vi "CoilConfig.vi"(0 "Card Info":cluster{"Card Handle":u32, "Error Code":u32}, 1 "AO Channels":i32, 2 "Stop angle [deg]":dbl=8.0 min=0.75 max=16.7 step=0.01 format="%.2g", 5 "Frequency (Hz)":dbl, 7 "Field [mT]":dbl=8.0 min=0.75 max=16.7 step=0.01 format="%.2g", 9 "Bit Resolution":i32, 11 "Clamp field [%]":sgl, 12 "Number of Turns":dbl) -> ()   [LabVIEW 2011]
uses:
  spcm_library/spcm_card.llb/setup DO/AO trigger.vi
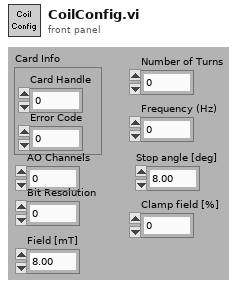
[diagram p1: front panel]
types:
  T1 = cluster{"Enable":bool, "Offs":i32, "Gain":i32, "Filter":i32, "Output Mode":u16}
  T2 = cluster{"Trig Termination":bool, "Trigger Source":u16, "External Trigger":u16, "Ext Pw":u32, "Trigger Delay (Samples)":u32, "Trig Output":bool}
  T3 = cluster{"Mode":u16, "Mem":u32, "Seg":u32, "Loop":u32}
  T4 = cluster{"Clock Mode":u16, "Sampling Rate (kHz)":i32, "Reference Clock (kHz)":i32, "Clock Output":bool, "Clock Termination":bool, "External Divider":i32}
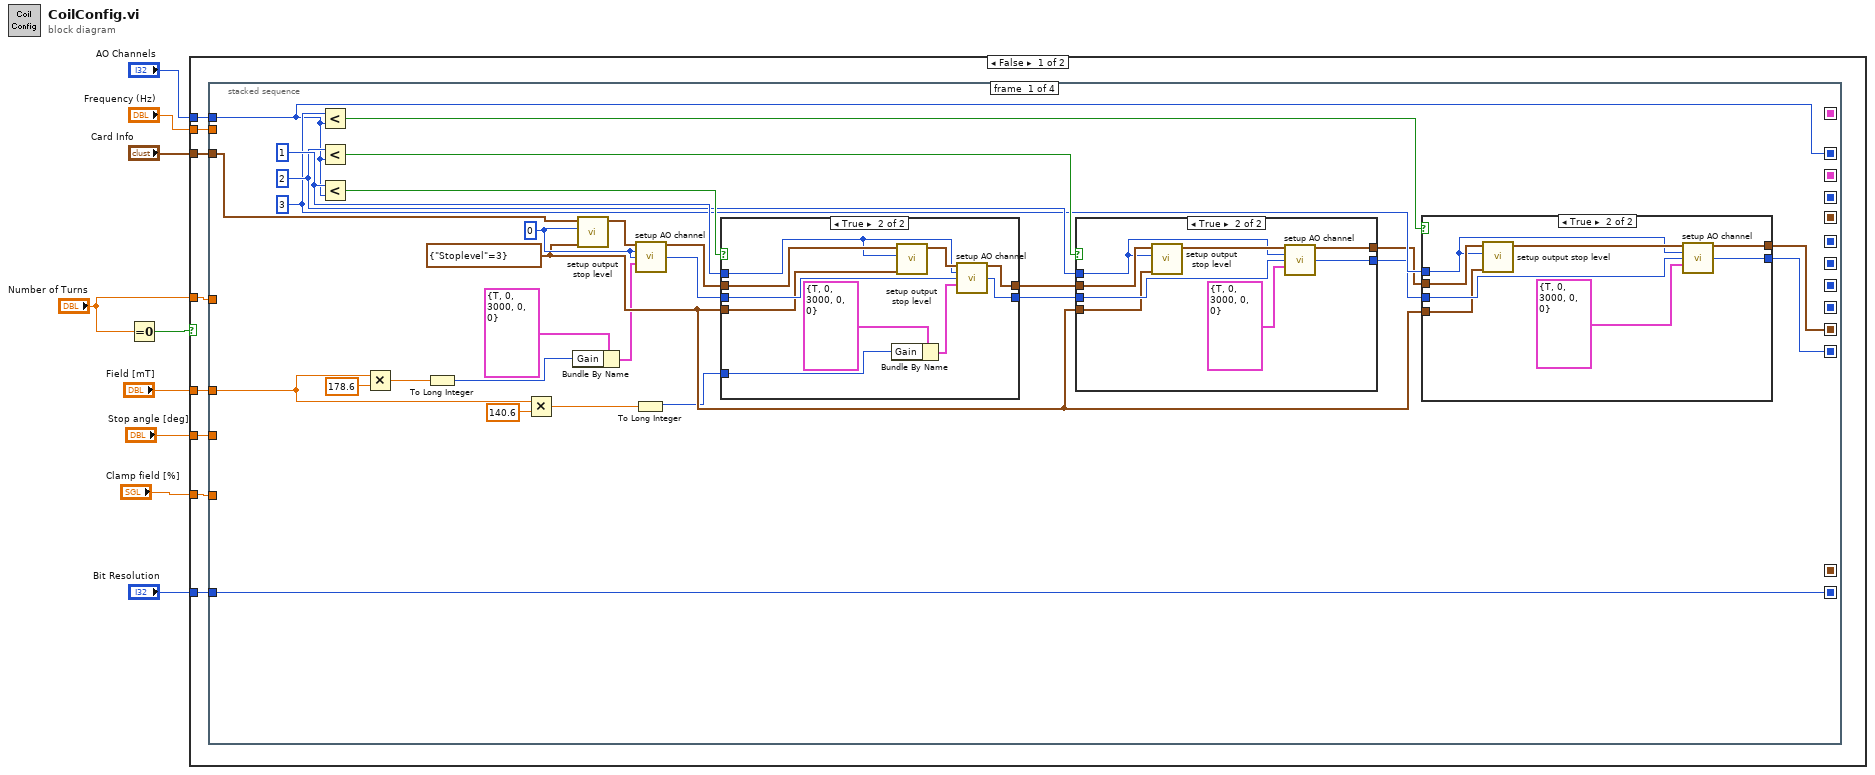
[diagram p0: block diagram]
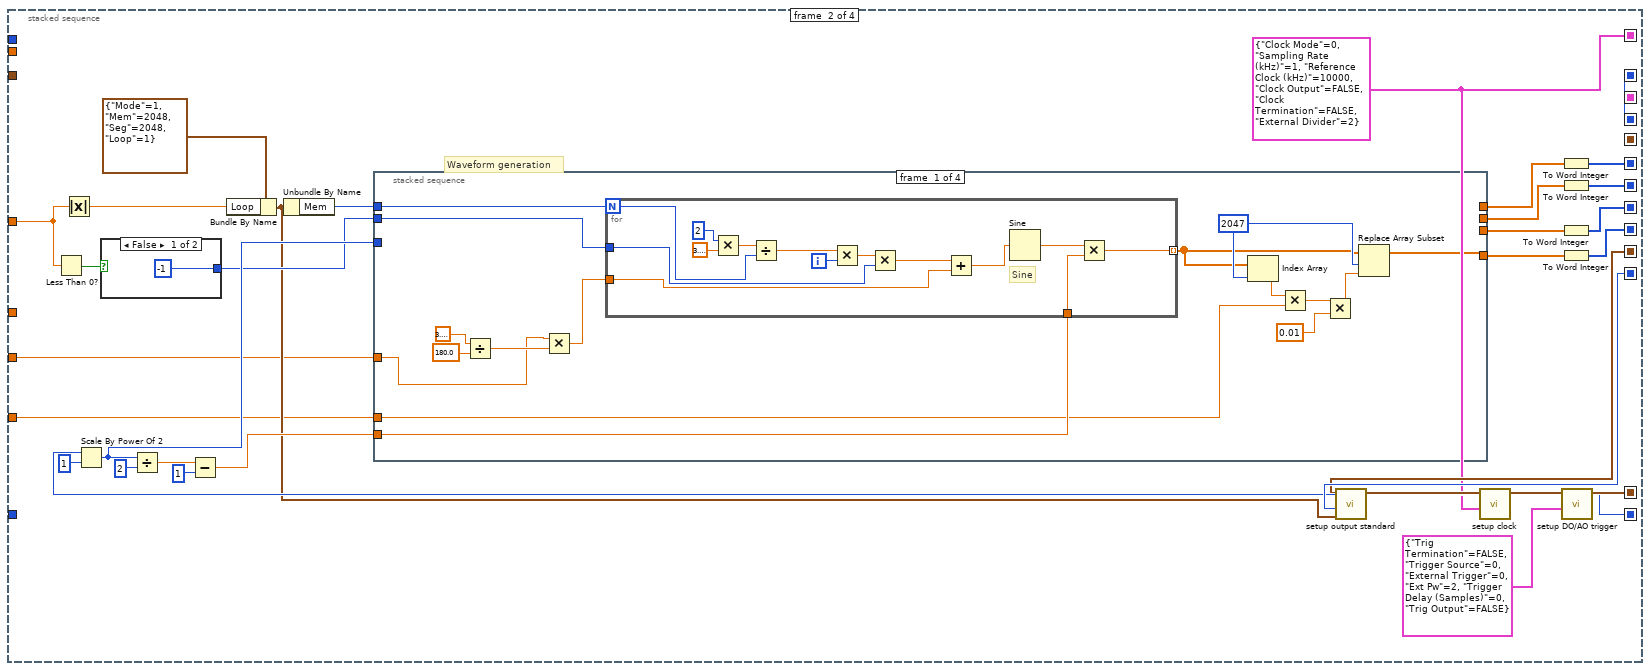
[diagram p5: hidden frame]
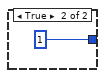
[diagram p6: hidden frame]
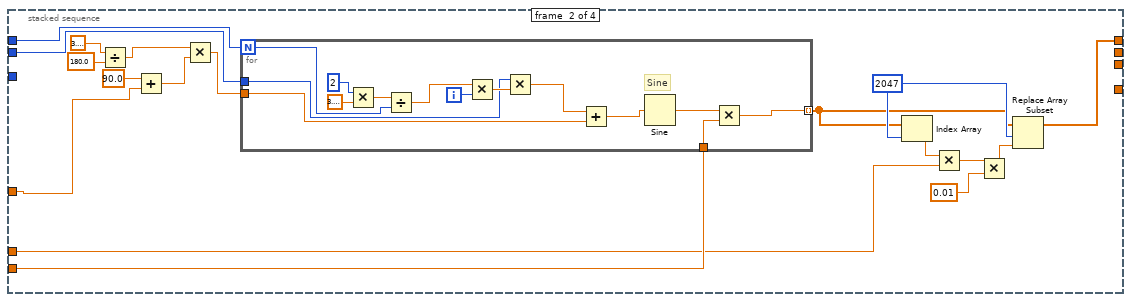
[diagram p7: hidden frame]
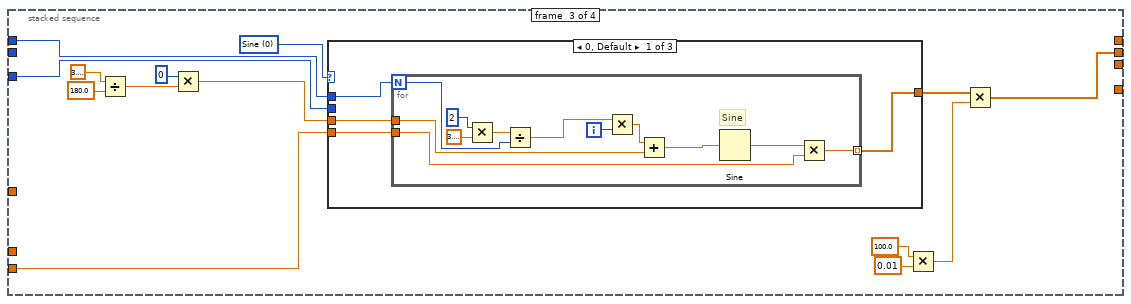
[diagram p8: hidden frame]
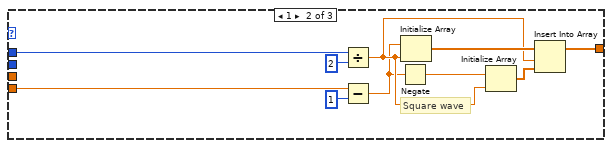
[diagram p9: hidden frame]
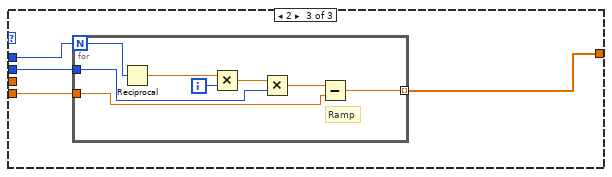
[diagram p10: hidden frame]
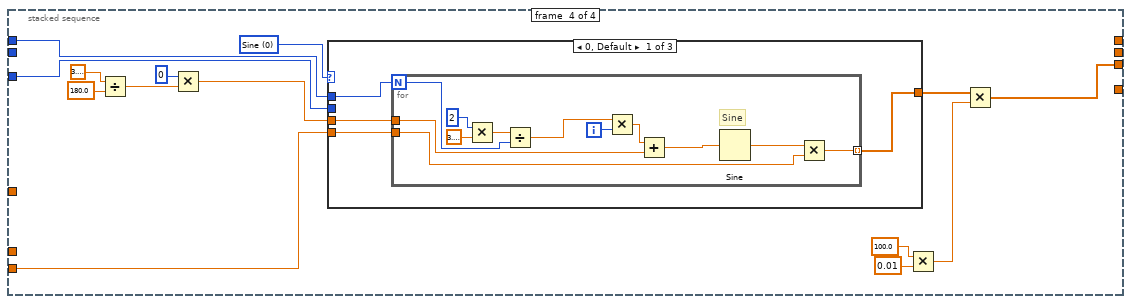
[diagram p11: hidden frame]
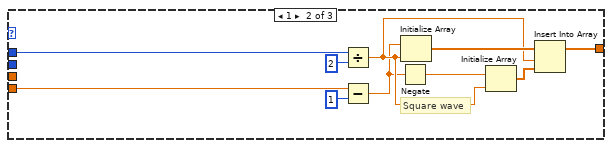
[diagram p12: hidden frame]
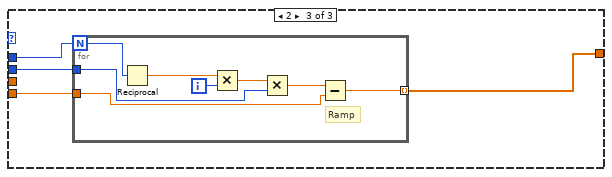
[diagram p13: hidden frame]
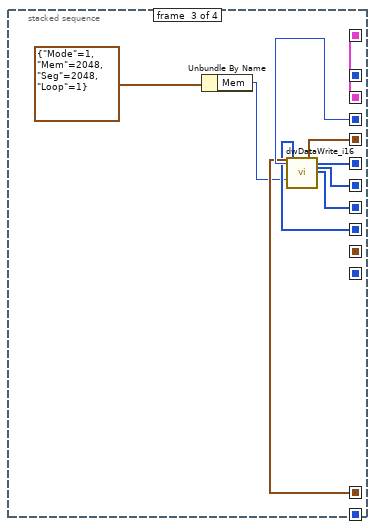
[diagram p14: hidden frame]
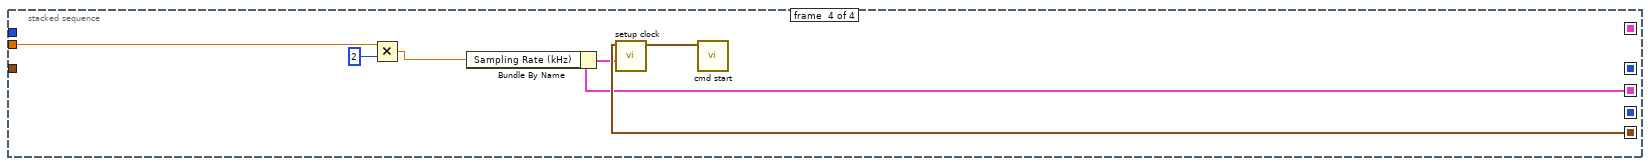
[diagram p15: hidden frame]
diagram:
  n1 = Equal To 0?(x="Number of Turns") -> (x = 0?=w3:bool)
  n2 = case shown="False" w3 {
    tunnel: "Frequency (Hz)" -> [w17 _]
    tunnel: "Clamp field [%]" -> [w16 _]
    tunnel: "Card Info" -> [w15 _]
    tunnel: "Number of Turns" -> [w14 _]
    tunnel: "Bit Resolution" -> [w13 _]
    tunnel: "AO Channels" -> [w12 _]
    tunnel: "Field [mT]" -> [w11 _]
    tunnel: "Stop angle [deg]" -> [w10 _]
    frame False {
      n3 = stacked-sequence {
        seq-local: [w29 _ _ _] -> [_ w104 _ _]
        seq-local: [w31 _ _ _] -> [_ w84 _ _]
        seq-local: [w44 _ _ _] -> [_ w102 _ _]
        seq-local: [w30 _ _ _] -> [_ w106 _ _]
        seq-local: [_ w88 _ _] -> [_ _ w280 _]
        seq-local: [_ w84 _ _] -> [_ _ w288 _]
        seq-local: [_ w108 _ _] -> [_ _ w287 _]
        seq-local: [_ w100 _ _] -> [_ _ w283 _]
        seq-local: [_ w99 _ _] -> [_ _ w284 _]
        seq-local: [_ w98 _ _] -> [_ _ w285 _]
        seq-local: [_ w97 _ _] -> [_ _ w286 _]
        seq-local: [_ _ w281 _] -> [_ _ _ w294]
        seq-local: [_ _ w280 _] -> [_ _ _ w293]
        tunnel: w13 -> [w29 _ _ _]
        tunnel: w12 -> [w31 _ _ _]
        tunnel: w15 -> [w28 _ _ _]
        tunnel: w16 -> [_ w83 _ _]
        tunnel: w14 -> [_ w81 _ _]
        tunnel: w17 -> [_ _ _ w290]
        tunnel: w11 -> [w18 _ _ _]
        tunnel: w10 -> [_ w79 _ _]
        frame #0 {
          w23 = cluster{"Stoplevel":u16} {"Stoplevel"=3} ("Stop Level")
          w36 = 3
          w38 = 2
          w45 = 1
          w42 = 0
          n4 = Less?(x=w36, y=w31) -> (x < y?=w37:bool)
          n5 = Less?(x=w38, y=w31) -> (x < y?=w39:bool)
          n6 = Less?(x=w45, y=w31) -> (x < y?=w46:bool)
          n7 = Multiply(x=w18, y=178.6) -> (x*y=w26:dbl)
          n8 = To Long Integer(number=w26) -> (32bit integer=w20:i32)
          n9 = Multiply(x=w18, y=140.6) -> (x*y=w25:dbl)
          n10 = Bundle By Name(cluster=T1 {"Enable"=TRUE, "Offs"=0, "Gain"=3000, "Filter"=0, "Output Mode"=0} ("Input Channel Settings"), "Gain"=w20) -> (w21:T1)
          n11 = call "setup output stop level.vi"("Stop Level"=w23, "Index"=w42, "Card Info In"=w28) -> ("Card Info Out"=w43:cluster{"Card Handle":u32, "Error Code":u32})  [unwired: 4 in]
          n12 = To Long Integer(number=w25) -> (32bit integer=w19:i32)
          n13 = call "setup AO channel.vi"("Card Info In"=w43, "Channel Index"=w42, "Channel Mask In"=w42, "Input Channel Settings"=w21) -> ("Card Info Out"=w41:cluster{"Card Handle":u32, "Error Code":u32}, "Channel MaskOut"=w40:i32)  [unwired: 10 in]
          n14 = case shown="True" w46 {
            tunnel: [w68 w76] -> w35
            tunnel: w41 -> [w68 w78]
            tunnel: w45 -> [_ w74]
            tunnel: w40 -> [w67 w75]
            tunnel: w23 -> [_ w73]
            tunnel: [w67 w72] -> w33
            tunnel: w19 -> [_ w69]
            frame False {
            }
            frame True {
              n15 = Bundle By Name(cluster=T1 {"Enable"=TRUE, "Offs"=0, "Gain"=3000, "Filter"=0, "Output Mode"=0} ("Input Channel Settings 2"), "Gain"=w69) -> (w71:T1)
              n16 = call "setup output stop level.vi"("Stop Level"=w73, "Index"=w74, "Card Info In"=w78) -> ("Card Info Out"=w77:cluster{"Card Handle":u32, "Error Code":u32})  [unwired: 4 in]
              n17 = call "setup AO channel.vi"("Card Info In"=w77, "Channel Index"=w74, "Channel Mask In"=w75, "Input Channel Settings"=w71) -> ("Card Info Out"=w76:cluster{"Card Handle":u32, "Error Code":u32}, "Channel MaskOut"=w72:i32)  [unwired: 10 in]
            }
          }
          n18 = case shown="True" w39 {
            tunnel: [w58 w64] -> w34
            tunnel: w35 -> [w58 w66]
            tunnel: w38 -> [_ w62]
            tunnel: w33 -> [w57 w63]
            tunnel: w23 -> [_ w61]
            tunnel: [w57 w60] -> w32
            frame False {
            }
            frame True {
              n19 = call "setup output stop level.vi"("Stop Level"=w61, "Index"=w62, "Card Info In"=w66) -> ("Card Info Out"=w65:cluster{"Card Handle":u32, "Error Code":u32})  [unwired: 4 in]
              n20 = call "setup AO channel.vi"("Card Info In"=w65, "Channel Index"=w62, "Channel Mask In"=w63, "Input Channel Settings"=T1 {"Enable"=TRUE, "Offs"=0, "Gain"=3000, "Filter"=0, "Output Mode"=0} ("Input Channel Settings 3")) -> ("Card Info Out"=w64:cluster{"Card Handle":u32, "Error Code":u32}, "Channel MaskOut"=w60:i32)  [unwired: 10 in]
            }
          }
          n21 = case shown="True" w37 {
            tunnel: [w48 w54] -> w44
            tunnel: w34 -> [w48 w56]
            tunnel: w36 -> [_ w52]
            tunnel: w32 -> [w47 w53]
            tunnel: w23 -> [_ w51]
            tunnel: [w47 w50] -> w30
            frame False {
            }
            frame True {
              n22 = call "setup output stop level.vi"("Stop Level"=w51, "Index"=w52, "Card Info In"=w56) -> ("Card Info Out"=w55:cluster{"Card Handle":u32, "Error Code":u32})  [unwired: 4 in]
              n23 = call "setup AO channel.vi"("Card Info In"=w55, "Channel Index"=w52, "Channel Mask In"=w53, "Input Channel Settings"=T1 {"Enable"=TRUE, "Offs"=0, "Gain"=3000, "Filter"=0, "Output Mode"=0} ("Input Channel Settings 4")) -> ("Card Info Out"=w54:cluster{"Card Handle":u32, "Error Code":u32}, "Channel MaskOut"=w50:i32)  [unwired: 10 in]
            }
          }
        }
        frame #1 {
          w88 = T4 {"Clock Mode"=0, "Sampling Rate (kHz)"=1, "Reference Clock (kHz)"=10000, "Clock Output"=FALSE, "Clock Termination"=FALSE, "External Divider"=2} ("Clock Settings")
          # "Waveform generation"
          n24 = Less Than 0?(x=w81) -> (x < 0?=w82:bool)
          n25 = Absolute Value(x=w81) -> (abs(x)=w80:dbl)
          n26 = Scale By Power Of 2(n=w104, x=1) -> (x*2^n=w89:i32)
          n27 = case shown="False" w82 {
            tunnel: [i16 -1 ("Phase 3") i16 1 ("Phase 3")] -> w87
            frame False {
            }
            frame True {
            }
          }
          n28 = Divide(x=w89, y=2) -> (x/y=w90:dbl)
          n29 = Subtract(x=w90, y=1) -> (x-y=w92:dbl)
          n30 = Bundle By Name(cluster=T3 {"Mode"=1, "Mem"=2048, "Seg"=2048, "Loop"=1} ("Mode Setup"), "Loop"=w80) -> (w85:T3)
          n31 = Unbundle By Name(w85) -> ("Mem"=w103:u32)
          n32 = stacked-sequence {
            tunnel: [w115 _ _ _] -> w101
            tunnel: w103 -> [w128 w160 w182 w234]
            tunnel: [_ w145 _ _] -> w96
            tunnel: [_ _ w185 _] -> w95
            tunnel: [_ _ _ w237] -> w94
            tunnel: w92 -> [w127 w159 w181 w233]
            tunnel: w89 -> [_ _ w180 w232]
            tunnel: w87 -> [w122 w155 _ _]
            tunnel: w83 -> [w113 w143 _ _]
            tunnel: w79 -> [w121 w151 _ _]
            frame #0 {
              w120 = 2047 ("index")
              n33 = Divide(x=3.141592653589793, y=sgl 180.0 ("Numeric")) -> (x/y=w124:dbl)
              n34 = Multiply(x=w121, y=w124) -> (x*y=w123:dbl)
              n35 = for {
                N: w128 -> [w136]
                tunnel: [w132] -> w114 mode=indexing
                tunnel: w127 -> [w141]
                tunnel: w123 -> [w134]
                tunnel: w122 -> [w129]
                i -> [w137]
                # "Sine"
                n36 = Multiply(x=2, y=3.141592653589793) -> (x*y=w135:dbl)
                n37 = Divide(x=w135, y=w136) -> (x/y=w138:dbl)
                n38 = Multiply(x=w138, y=w137) -> (x*y=w131:dbl)
                n39 = Multiply(x=w131, y=w129) -> (x*y=w130:dbl)
                n40 = Add(x=w130, y=w134) -> (x+y=w133:dbl)
                n41 = Sine(x=w133) -> (sin(x)=w142:dbl)
                n42 = Multiply(x=w142, y=w141) -> (x*y=w132:dbl)
              }
              n43 = Index Array(array=w114, index=w120) -> (element=w116:dbl)
              n44 = Multiply(x=w116, y=w113) -> (x*y=w119:dbl)
              n45 = Multiply(x=w119, y=0.01) -> (x*y=w117:dbl)
              n46 = Replace Array Subset(array=w114, new element=w117, index=w120) -> (w115:dbl[])
            }
            frame #1 {
              w150 = 2047 ("index")
              n47 = Divide(x=3.141592653589793, y=sgl 180.0 ("Numeric")) -> (x/y=w154:dbl)
              n48 = Add(x=90.0, y=w151) -> (x+y=w153:dbl)
              n49 = Multiply(x=w154, y=w153) -> (x*y=w156:dbl)
              n50 = for {
                N: w160 -> [w168]
                tunnel: [w166] -> w144 mode=indexing
                tunnel: w159 -> [w173]
                tunnel: w156 -> [w164]
                tunnel: w155 -> [w161]
                i -> [w169]
                # "Sine"
                n51 = Multiply(x=2, y=3.141592653589793) -> (x*y=w167:dbl)
                n52 = Divide(x=w167, y=w168) -> (x/y=w170:dbl)
                n53 = Multiply(x=w170, y=w169) -> (x*y=w162:dbl)
                n54 = Multiply(x=w161, y=w162) -> (x*y=w163:dbl)
                n55 = Add(x=w163, y=w164) -> (x+y=w165:dbl)
                n56 = Sine(x=w165) -> (sin(x)=w174:dbl)
                n57 = Multiply(x=w174, y=w173) -> (x*y=w166:dbl)
              }
              n58 = Index Array(array=w144, index=w150) -> (element=w146:dbl)
              n59 = Multiply(x=w146, y=w143) -> (x*y=w149:dbl)
              n60 = Multiply(x=w149, y=0.01) -> (x*y=w147:dbl)
              n61 = Replace Array Subset(array=w144, new element=w147, index=w150) -> (w145:dbl[])
            }
            frame #2 {
              w183 = u16 0 items=["Sine", "Square", "Ramp"] ("Waveform 3")
              n62 = Divide(x=3.141592653589793, y=sgl 180.0 ("Numeric")) -> (x/y=w177:dbl)
              n63 = Multiply(x=i16 0 ("Phase"), y=w177) -> (x*y=w176:dbl)
              n64 = case shown="0, Default" w183 {
                tunnel: w182 -> [w192 w214 w218]
                tunnel: [w191 w210 w217] -> w184
                tunnel: w181 -> [w190 w205 w216]
                tunnel: w180 -> [_ _ w215]
                tunnel: w176 -> [w189 _ _]
                frame 0, Default {
                  n65 = for {
                    N: w192 -> [w198]
                    tunnel: [w196] -> w191 mode=indexing
                    tunnel: w190 -> [w203]
                    tunnel: w189 -> [w193]
                    i -> [w199]
                    # "Sine"
                    n66 = Multiply(x=2, y=3.141592653589793) -> (x*y=w197:dbl)
                    n67 = Divide(x=w197, y=w198) -> (x/y=w200:dbl)
                    n68 = Multiply(x=w200, y=w199) -> (x*y=w194:dbl)
                    n69 = Add(x=w194, y=w193) -> (x+y=w195:dbl)
                    n70 = Sine(x=w195) -> (sin(x)=w204:dbl)
                    n71 = Multiply(x=w204, y=w203) -> (x*y=w196:dbl)
                  }
                }
                frame 1 {
                  # "Square wave"
                  n72 = Divide(x=w214, y=2) -> (x/y=w209:dbl)
                  n73 = Subtract(x=w205, y=1) -> (x-y=w207:dbl)
                  n74 = Negate(x=w207) -> (-x=w208:dbl)
                  n75 = Initialize Array(w207, w209) -> (w212:dbl[])
                  n76 = Initialize Array(w208, w209) -> (w211:dbl[])
                  n77 = Insert Into Array(array=w212, index=w209, new element=w211) -> (w210:dbl[])
                }
                frame 2 {
                  n78 = for {
                    N: w218 -> [w221]
                    tunnel: [w223] -> w217 mode=indexing
                    tunnel: w216 -> [w220]
                    tunnel: w215 -> [w219]
                    i -> [w225]
                    # "Ramp"
                    n79 = Reciprocal(x=w221) -> (1/x=w226:dbl)
                    n80 = Multiply(x=w226, y=w225) -> (x*y=w224:dbl)
                    n81 = Multiply(x=w224, y=w219) -> (x*y=w222:dbl)
                    n82 = Subtract(x=w222, y=w220) -> (x-y=w223:dbl)
                  }
                }
              }
              n83 = Multiply(x=sgl 100.0 ("Ampl"), y=0.01) -> (x*y=w186:dbl)
              n84 = Multiply(x=w184, y=w186) -> (x*y=w185:dbl[])
            }
            frame #3 {
              w236 = u16 0 items=["Sine", "Square", "Ramp"] ("Waveform 4")
              n85 = Divide(x=3.141592653589793, y=sgl 180.0 ("Numeric")) -> (x/y=w230:dbl)
              n86 = Multiply(x=i16 0 ("Phase"), y=w230) -> (x*y=w227:dbl)
              n87 = case shown="0, Default" w236 {
                tunnel: w234 -> [w244 w266 w270]
                tunnel: [w243 w262 w269] -> w235
                tunnel: w233 -> [w242 w257 w268]
                tunnel: w232 -> [_ _ w267]
                tunnel: w227 -> [w241 _ _]
                frame 0, Default {
                  n88 = for {
                    N: w244 -> [w250]
                    tunnel: [w248] -> w243 mode=indexing
                    tunnel: w242 -> [w255]
                    tunnel: w241 -> [w245]
                    i -> [w251]
                    # "Sine"
                    n89 = Multiply(x=2, y=3.141592653589793) -> (x*y=w249:dbl)
                    n90 = Divide(x=w249, y=w250) -> (x/y=w252:dbl)
                    n91 = Multiply(x=w252, y=w251) -> (x*y=w247:dbl)
                    n92 = Add(x=w247, y=w245) -> (x+y=w246:dbl)
                    n93 = Sine(x=w246) -> (sin(x)=w256:dbl)
                    n94 = Multiply(x=w256, y=w255) -> (x*y=w248:dbl)
                  }
                }
                frame 1 {
                  # "Square wave"
                  n95 = Divide(x=w266, y=2) -> (x/y=w261:dbl)
                  n96 = Subtract(x=w257, y=1) -> (x-y=w259:dbl)
                  n97 = Negate(x=w259) -> (-x=w260:dbl)
                  n98 = Initialize Array(w259, w261) -> (w264:dbl[])
                  n99 = Initialize Array(w260, w261) -> (w263:dbl[])
                  n100 = Insert Into Array(array=w264, index=w261, new element=w263) -> (w262:dbl[])
                }
                frame 2 {
                  n101 = for {
                    N: w270 -> [w273]
                    tunnel: [w275] -> w269 mode=indexing
                    tunnel: w268 -> [w272]
                    tunnel: w267 -> [w271]
                    i -> [w277]
                    # "Ramp"
                    n102 = Reciprocal(x=w273) -> (1/x=w278:dbl)
                    n103 = Multiply(x=w278, y=w277) -> (x*y=w276:dbl)
                    n104 = Multiply(x=w276, y=w271) -> (x*y=w274:dbl)
                    n105 = Subtract(x=w274, y=w272) -> (x-y=w275:dbl)
                  }
                }
              }
              n106 = Multiply(x=sgl 100.0 ("Amp"), y=0.01) -> (x*y=w238:dbl)
              n107 = Multiply(x=w235, y=w238) -> (x*y=w237:dbl[])
            }
          }
          n108 = call "setup output standard.vi"("Mode Setup"=w85, "Channel Mask Low"=w106, "Card Info In"=w102) -> ("Card Info Out"=w109:cluster{"Card Handle":u32, "Error Code":u32})  [unwired: 4 in]
          n109 = call "setup clock.vi"("Clock Settings"=w88, "Card Info In"=w109) -> ("Card Info Out"=w110:cluster{"Card Handle":u32, "Error Code":u32})  [unwired: 4 in, 1 out]
          n110 = To Word Integer(number=w96) -> (16bit integer=w98:i16[])
          n111 = To Word Integer(number=w95) -> (16bit integer=w99:i16[])
          n112 = To Word Integer(number=w94) -> (16bit integer=w100:i16[])
          n113 = To Word Integer(number=w101) -> (16bit integer=w97:i16[])
          n114 = call "setup DO/AO trigger.vi"("Trigger Settings"=T2 {"Trig Termination"=FALSE, "Trigger Source"=0, "External Trigger"=0, "Ext Pw"=2, "Trigger Delay (Samples)"=0, "Trig Output"=FALSE}, "Card Info In"=w110) -> ("Card Info Out"=w108:cluster{"Card Handle":u32, "Error Code":u32})  [unwired: 4 in, 1 out]
        }
        frame #2 {
          n115 = Unbundle By Name(T3 {"Mode"=1, "Mem"=2048, "Seg"=2048, "Loop"=1} ("Mode Setup")) -> ("Mem"=w282:u32)
          n116 = call "dwDataWrite_i16.vi"("Card Info In"=w287, "Channel Count"=w288, "Length (Samples per Channel)"=w282, "Ch 0"=w286, "Ch 1"=w285, "Ch 2"=w284, "Ch 3"=w283) -> ("Card Info Out"=w281:cluster{"Card Handle":u32, "Error Code":u32})  [unwired: 20 in]
        }
        frame #3 {
          n117 = Multiply(x=w290, y=2) -> (x*y=w291:dbl)
          n118 = Bundle By Name(cluster=w293, "Sampling Rate (kHz)"=w291) -> (w292:T4)
          n119 = call "setup clock.vi"("Clock Settings"=w292, "Card Info In"=w294) -> ("Card Info Out"=w295:cluster{"Card Handle":u32, "Error Code":u32})  [unwired: 4 in, 1 out]
          n120 = call "cmd start.vi"("Card Info In"=w295) -> ()  [unwired: 6 in, 1 out]
        }
      }
    }
    frame True {
    }
  }
